vi "Close_H5_file.vi"(8 "error in (no error)":errorcluster, 11 "ref":i32) -> (0 "error out":errorcluster)   [LabVIEW 2012]
uses:
  <vilib>/addons/h5labview/H5File.lvlib
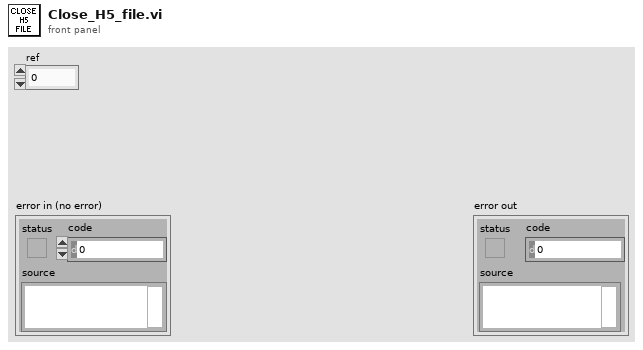
[diagram p1: front panel]
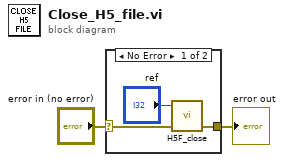
[diagram p0: block diagram]
diagram:
  n1 = case shown="No Error" "error in (no error)" {
    selector: "error in (no error)" -> [w5 w6]
    tunnel: [w4 w6] -> w1
    frame No Error {
      n2 = call <vilib>:"H5F_close.vi"("error in (no error)"=w5, "ref"="ref") -> ("error out"=w4:errorcluster)  [unwired: 3 in]
    }
    frame Error {
    }
  }
  "error out" <- w1
